vi "ex_GetData.vi"(0 "channel info in":T3[](array[typedef]) {"Delta X" format="%.2p"; "X0" format="%<%X\n%x>T"; "Timestamp" format="%<%X\n%x>T"}, 1 "chunk in":string, 2 "# of samples to read (all: -1)":i32=-1, 3 "file refs in":T1, 4 "# of samples read":i32, 5 "delimiter":string, 6 "# of samples in channel group":i32, 7 "error in":errorcluster, 8 "Decimal Separator":string, 9 "file_params":T2 {"time preference" items=["Absolute", "Relative"]; "x_columns" items=["None", "One", "Multiple"]}, 15 "first_packet?":bool, 17 "origin timestamp":timestamp format="%<%X\n%x>T", 27 "relative time?":bool) -> (14 "end-of-file?":bool, 16 "Comment":string, 20 "channel info out":T3[](array[typedef]) {"Delta X" format="%.2p"; "X0" format="%<%X\n%x>T"; "Timestamp" format="%<%X\n%x>T"}, 21 "chunk remainder":string, 22 "Samples read out":u32, 23 "file refs out":T1={"file ref"=refnum, "file size (bytes:0)"=0, "read pointer (bytes:0)"=0, "chunk size (bytes:65000)"=65000}, 24 "Signals":waveform(dbl)[](array[waveform]), 25 "error out":errorcluster, 26 "read segment header":bool)   [LabVIEW 2017]
uses:
  <vilib>/express/express shared/ExFile.llb/ex_AllChanInfo.ctl
  <vilib>/express/express shared/ExFile.llb/ex_FileReference.ctl
  <vilib>/express/express input/ExFileReadBlock.llb/ex_ReadFileParams.ctl
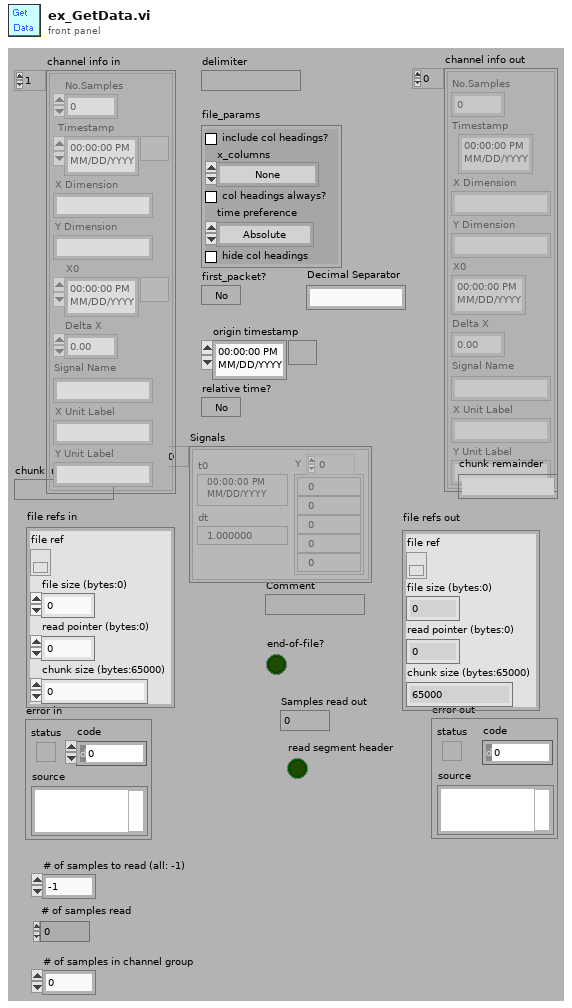
[diagram p1: front panel]
types:
  T1 = typedef "ex_FileReference.ctl" = cluster{"file ref":refnum<file>, "file size (bytes:0)":i32, "read pointer (bytes:0)":i32, "chunk size (bytes:65000)":i32}
  T2 = typedef "ex_ReadFileParams.ctl" = cluster{"include col headings?":bool, "x_columns":u16, "col headings always?":bool, "time preference":u16, "hide col headings":bool}
  T3 = typedef "ex_AllChanInfo.ctl" = cluster{"No.Samples":i32, "Timestamp":timestamp, "X Dimension":string, "Y Dimension":string, "X0":timestamp, "Delta X":dbl, "Signal Name":string, "X Unit Label":string, "Y Unit Label":string}
  T4 = typedef "ex_WaveformAttribsPlus.ctl" = cluster{"Start Timestamp":timestamp, "Timestamp":timestamp, "Relative Time?":bool, "X Dimension":string, "Signal Name":string, "Y Units":string, "X0":timestamp, "dX":dbl, "nPoints":i32}
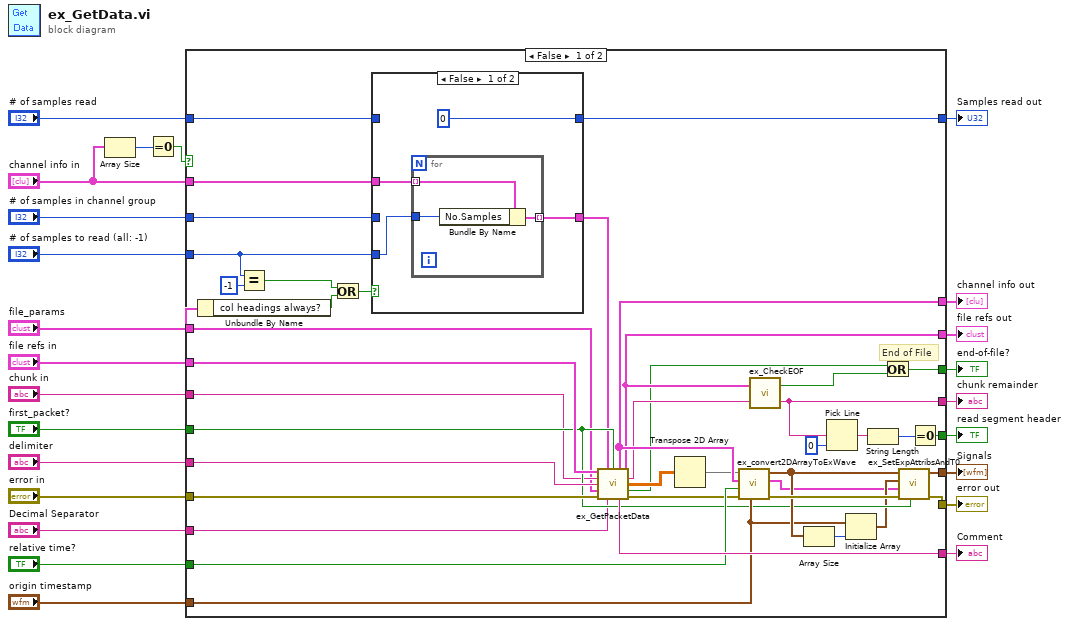
[diagram p0: block diagram]
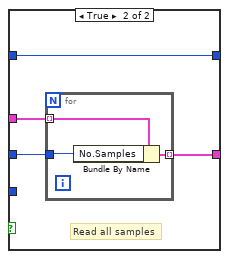
[diagram p2: hidden frame]
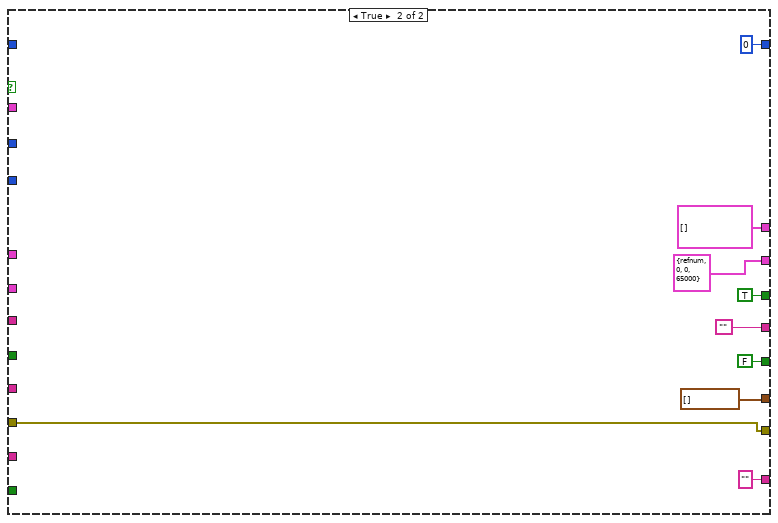
[diagram p3: hidden frame]
diagram:
  n1 = Array Size(array="channel info in") -> (size(s)=w2:i32)
  n2 = Equal To 0?(x=w2) -> (x = 0?=w1:bool)
  n3 = case shown="False" w1 {
    tunnel: [w65 "" ("comment")] -> w24
    tunnel: [w64 T3[] [] ("channel info out")] -> w23
    tunnel: "relative time?" -> [w63 _]
    tunnel: [w62 waveform(dbl)[] [] ("Signals With Attributes")] -> w21
    tunnel: "file refs in" -> [w61 _]
    tunnel: "error in" -> [w60 w81]
    tunnel: "delimiter" -> [w59 _]
    tunnel: [w58 T1 {"file ref"=refnum, "file size (bytes:0)"=0, "read pointer (bytes:0)"=0, "chunk size (bytes:65000)"=65000} ("dup file refs")] -> w17
    tunnel: [w50 TRUE] -> w16
    tunnel: [w49 w81] -> w15
    tunnel: "origin timestamp" -> [w47 _]
    tunnel: "first_packet?" -> [w45 _]
    tunnel: "channel info in" -> [w42 _]
    tunnel: "# of samples in channel group" -> [w40 _]
    tunnel: "# of samples read" -> [w39 _]
    tunnel: [w38 u32 0 ("t")] -> w10
    tunnel: "chunk in" -> [w34 _]
    tunnel: [w33 FALSE] -> w8
    tunnel: [w32 ""] -> w7
    tunnel: "file_params" -> [w30 _]
    tunnel: "# of samples to read (all: -1)" -> [w26 _]
    tunnel: "Decimal Separator" -> [w25 _]
    frame False {
      # "End of File"
      n4 = Unbundle By Name(w30) -> ("col headings always?"=w28:bool)
      n5 = Equal?(x=w26, y=-1) -> (x = y?=w29:bool)
      n6 = Or(x=w29, y=w28) -> (x .or. y?=w27:bool)
      n7 = case shown="False" w27 {
        tunnel: w39 -> [_ w76]
        tunnel: w40 -> [_ w73]
        tunnel: [u32 0 ("t") w76] -> w38
        tunnel: w42 -> [w68 w75]
        tunnel: [w67 w74] -> w41
        tunnel: w26 -> [w66 _]
        frame False {
          n8 = for {
            tunnel: w68 -> [w72] mode=indexing
            tunnel: [w71] -> w67 mode=indexing
            tunnel: w66 -> [w70]
            n9 = Bundle By Name(cluster=w72, "No.Samples"=w70) -> (w71:T3)
          }
        }
        frame True {
          # "Read all samples"
          n10 = for {
            tunnel: w75 -> [w79] mode=indexing
            tunnel: [w78] -> w74 mode=indexing
            tunnel: w73 -> [w77]
            n11 = Bundle By Name(cluster=w79, "No.Samples"=w77) -> (w78:T3)
          }
        }
      }
      n12 = call <vilib>:"ex_GetPacketData.vi"("file refs"=w61, "channel info in"=w41, "first call?"=w45, "current chunk"=w34, "delimiter"=w59, "file_params"=w30, "error in (no error)"=w60, "Decimal Separator"=w25) -> ("channel info out"=w64:T3[], "dup file refs"=w58:T1, "chunk out"=w54:string, "data"=w57:dbl[][], "end-of-file?"=w53:bool, "comment"=w65:string, "error out"=w55:errorcluster)  [unwired: 1 out]
      n13 = Transpose 2D Array(2D array=w57) -> (transposed array=w51:dbl[][])
      n14 = call <vilib>:"ex_convert2DArrayToExWave.vi"("Origin Timestamp"=w47, "error in (no error)"=w55, "Relative Time?"=w63, "channel info"=w64, "Y Data"=w51) -> ("error out"=w56:errorcluster, "Express Attributes"=w43:T4[], "Signals"=w48:waveform(dbl)[])  [unwired: 4 out]
      n15 = call <vilib>:"ex_CheckEOF.vi"("chunk in"=w54, "file refs"=w58) -> ("chunk remainder"=w32:string, "EOF?"=w52:bool)
      n16 = Array Size(array=w48) -> (size(s)=w46:i32)
      n17 = Pick Line(multi-line string=w32, line index=0) -> (output string=w35:string)  [unwired: 1 out]
      n18 = Initialize Array(w47, w46) -> (w44:timestamp[])
      n19 = String Length(string=w35) -> (length=w37:i32)
      n20 = Or(x=w53, y=w52) -> (x .or. y?=w50:bool)
      n21 = call <vilib>:"ex_SetExpAttribsAndT0.vi"("Latch Origin TS? (T)"=w45, "error in (no error)"=w56, "Express Attributes Plus in"=w43, "Origin Timestamps"=w44, "Signals"=w48) -> ("error out"=w49:errorcluster, "Signals With Attributes"=w62:waveform(dbl)[])  [unwired: 1 in, 4 out]
      n22 = Equal To 0?(x=w37) -> (x = 0?=w33:bool)
    }
    frame True {
    }
  }
  "Comment" <- w24
  "channel info out" <- w23
  "error out" <- w15
  "Signals" <- w21
  "end-of-file?" <- w16
  "chunk remainder" <- w7
  "file refs out" <- w17
  "Samples read out" <- w10
  "read segment header" <- w8
